vi "Recursive Control Lookup.vi"(8 "error in (no error)":errorcluster, 9 "Tag":string, 10 "Cluster in":refnum<vi>, 11 "Lookup Table in":variant) -> (0 "error out":errorcluster, 3 "Lookup Table in":variant)   [LabVIEW 2015, in "State Accessor Scripter.lvclass"]
uses:
  State Accessor Scripter.lvclass
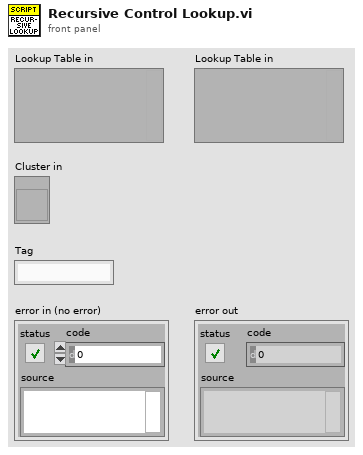
[diagram p1: front panel]
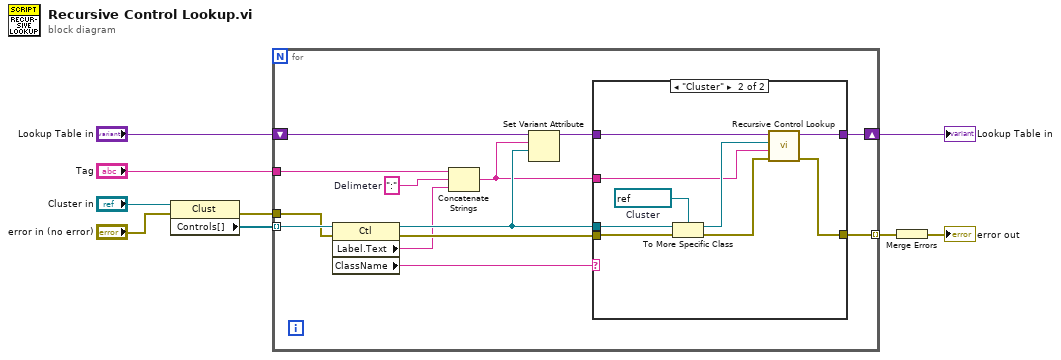
[diagram p0: block diagram]
diagram:
  n1 = property class="Clust"(reference="Cluster in", error in="error in (no error)") -> (error out=w5:errorcluster, "Controls[]"=w3:refnum<vi>[])  [unwired: 1 out]
  n2 = for {
    tunnel: w3 -> [w22] mode=indexing
    shift-right: [w11] -> w9
    shift-left: "Lookup Table in" -> [w17]
    tunnel: w5 -> [w20]
    tunnel: "Tag" -> [w12]
    tunnel: [w10] -> w2 mode=indexing
    w18 = ":"  # Delimeter
    n3 = property class="Ctl"(reference=w22, error in=w20) -> (reference out=w15:refnum<vi>, error out=w19:errorcluster, "Label.Text"=w14:string, "ClassName"=w21:string)
    n4 = Concatenate Strings(w12, w18, w14) -> (w13:string)
    n5 = Set Variant Attribute(Variant=w17, name=w13, value=w15) -> (Variant out=w16:variant)  [unwired: 1 in, 2 out]
    n6 = case shown="\"Cluster\"" w21 {
      tunnel: w15 -> [_ w31]
      tunnel: w16 -> [w24 w33]
      tunnel: w19 -> [w23 w28]
      tunnel: w13 -> [_ w27]
      tunnel: [w24 w32] -> w11
      tunnel: [w23 w25] -> w10
      frame Default {
      }
      frame "Cluster" {
        w29 = refnum<vi> refnum  # Cluster
        n7 = To More Specific Class(target class=w29, reference=w31, error in=w28) -> (specific class reference=w30:refnum<vi>, error out=w26:errorcluster)
        n8 = call "Recursive Control Lookup.vi"("error in (no error)"=w26, "Tag"=w27, "Cluster in"=w30, "Lookup Table in"=w33) -> ("error out"=w25:errorcluster, "Lookup Table in"=w32:variant)  [unwired: 6 in]
      }
    }
  }
  "Lookup Table in" <- w9
  n9 = Merge Errors(w2) -> (→"error out":errorcluster)
